vi "Read SSH.vi"(8 "Error In":errorcluster, 11 "SFTP File In":refnum<class "SFTP File.lvclass">) -> (0 "Error Out":errorcluster, 2 "SSH":refnum<class "SSH.lvclass">, 3 "SFTP File Out":refnum<class "SFTP File.lvclass">)   [LabVIEW 2018, in "Toolkit.lvlib" / "SFTP File.lvclass"]
uses:
  SFTP File.lvclass
  SSH/SSH.lvclass
  SFTP File.lvclass/SFTP File.ctl
  SFTP/SFTP.lvclass/SFTP.ctl
  Session/Session.lvclass/Session.ctl
  SFTP/SFTP.lvclass
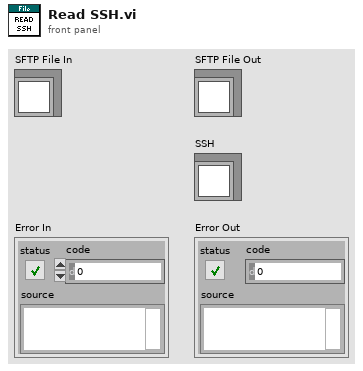
[diagram p1: front panel]
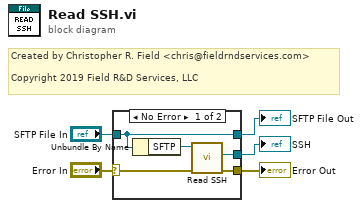
[diagram p0: block diagram]
diagram:
  # "Created by Christopher R. Field <chris@fieldrndservices.com>\n\nCopyright 2019 Field R&D Services, LLC"
  n1 = case shown="No Error" "Error In" {
    selector: "Error In" -> [w7 w12]
    tunnel: "SFTP File In" -> [w10 w11]
    tunnel: [w10 w11] -> w1
    tunnel: [w6 w12] -> w4
    tunnel: [w8 _] -> w3
    frame No Error {
      n2 = Unbundle By Name(w10) -> ("SFTP"=w9:refnum<class "SFTP.lvclass">)
      n3 = call "Read SSH.vi"("Error In"=w7, "SFTP In"=w9) -> ("Erorr Out"=w6:errorcluster, "SSH"=w8:refnum<class "SSH.lvclass">)  [unwired: 7 in, 1 out]
    }
    frame Error {
    }
  }
  "Error Out" <- w4
  "SSH" <- w3
  "SFTP File Out" <- w1
